vi "Manage Devices.vi"(0 "Devices queue":refnum<queue>, 1 "Table Ref In":refnum<vi>, 2 "DevNums In":i32[](array[numeric]), 3 "Col array in":refnum<class "Column.lvclass">[](array[class]), 4 "Table History ref":refnum<vi>, 5 "Layout ref":refnum<vi>) -> (7 "Devices queue out":refnum<queue>, 8 "Changes Made?":bool, 9 "DevNums Out":i32[](array[numeric]), 10 "Col array out":refnum<class "Column.lvclass">[](array[class]))   [LabVIEW 2013]
doc: "Add or Edit devices included in SetList table. Use this dialog to change SetList appearance (Column Name, Width, Colors) Trigger Line, Communication Port, etc...\nThis VI requires read/write access to Col array data."
uses:
  Device/Device.lvclass
  TypeDefs/AddDeviceRing.ctl
  ColumnVIs/Column/Column.lvclass
  TypeDefs/TableHistory.ctl
  TypeDefs/TableArray.ctl
  Master Device/Master Device.lvclass
panel:
  in  "Add Device":T1 items=["Select Type...", "DDS", "Novatech", "NI Card"]
  in  "Master Device Info":T2
  in  "Done":bool
  out "Device List in":refnum<class "Device.lvclass">[](array[class])
  in  "Slave Devices":T3(array[cluster])
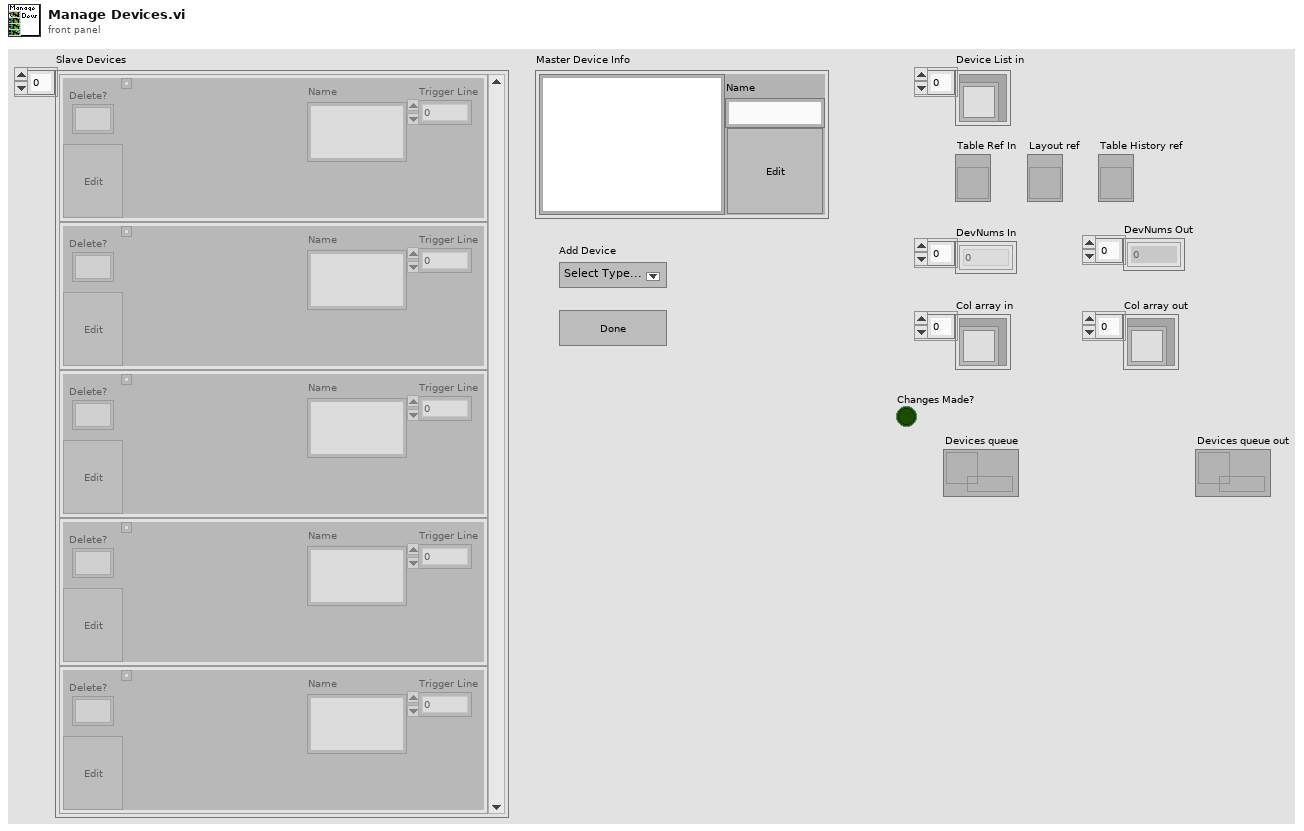
[diagram p1: front panel]
types:
  T1 = typedef "AddDeviceRing.ctl" = u16
  T2 = cluster{"2D Picture":picture, "Name":string, "Edit Device":bool}
  T3 = cluster{"Delete?":bool, "2D Picture":picture, "Name":string, "Trigger Line":i32, "Edit Device":bool}[]
  T4 = typedef "imagedata.ctl" = cluster{"image type":i32, "image depth":i32, "image":u8[], "mask":u8[], "colors":u32[], "Rectangle":cluster{"left":i16, "top":i16, "right":i16, "bottom":i16}}
  T5 = cluster{bool, "new picture":picture, "Name":string, "PB Trigger Line":u16, bool}
  T6 = cluster{"new picture":picture, "Name":string, bool}
  T7 = cluster{"Delete?":bool, "2D Picture":bool, "Name":bool, "Trigger Line":bool, "Edit Device":bool}[]
  T8 = cluster{"Delete?":bool, "2D Picture":picture, "Name":string, "Trigger Line":i32, "Edit Device":bool}
  T9 = cluster{"Delete?":bool, "new picture":picture, "Name":string, "Trigger Line":i32, "Edit Device":bool}[]
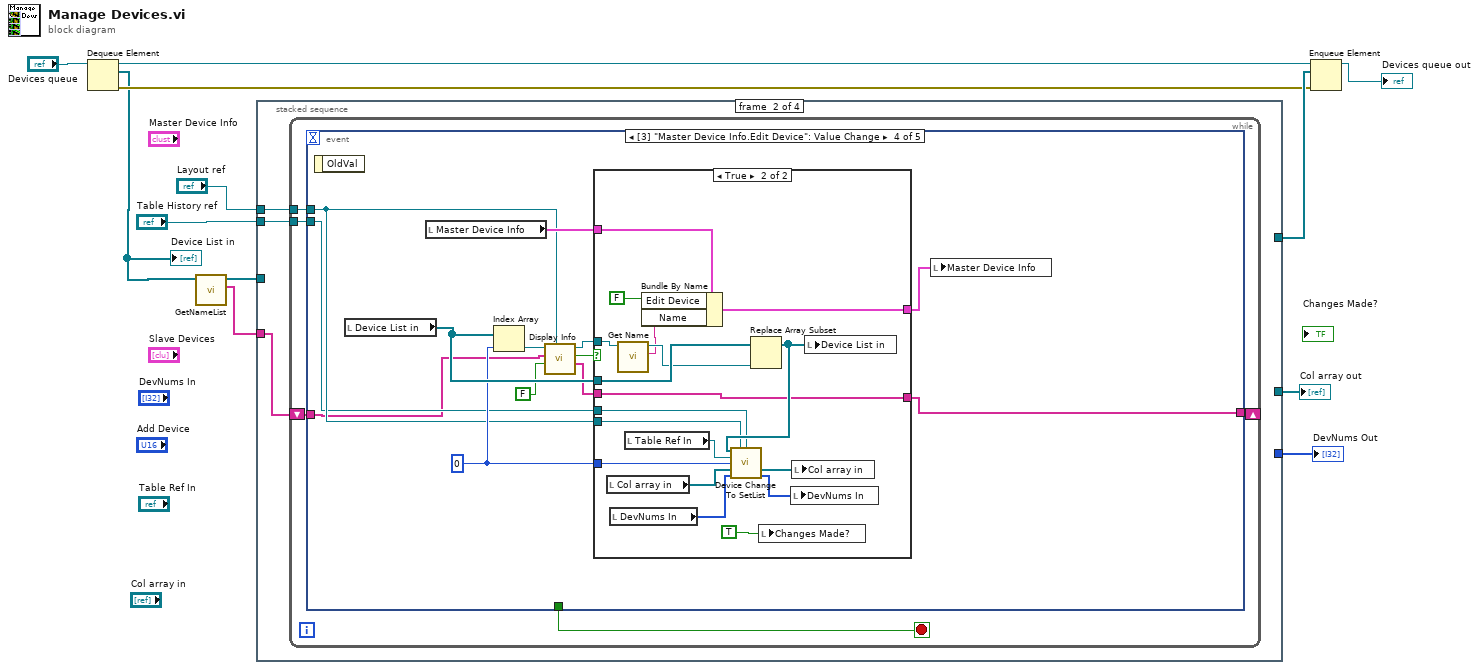
[diagram p0: block diagram]
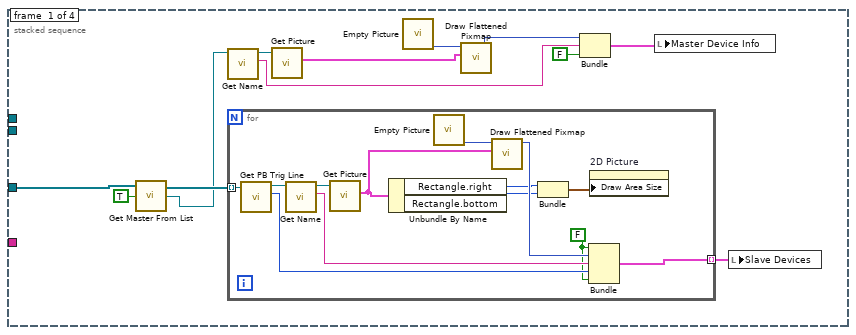
[diagram p2: hidden frame]
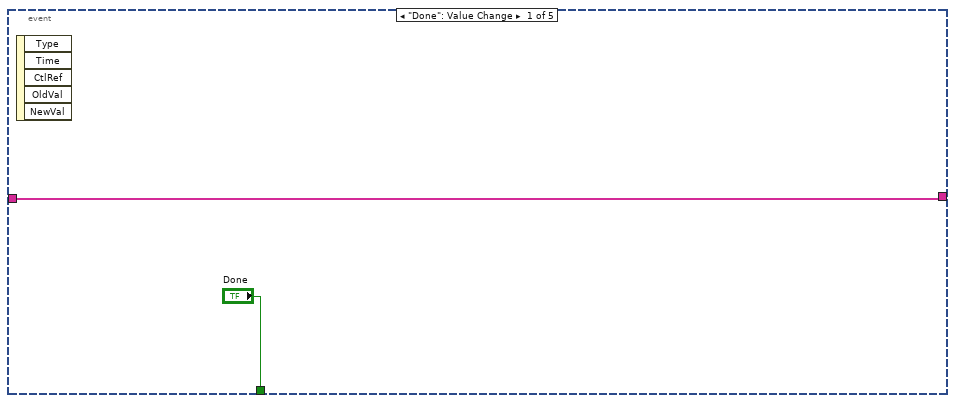
[diagram p3: hidden frame]
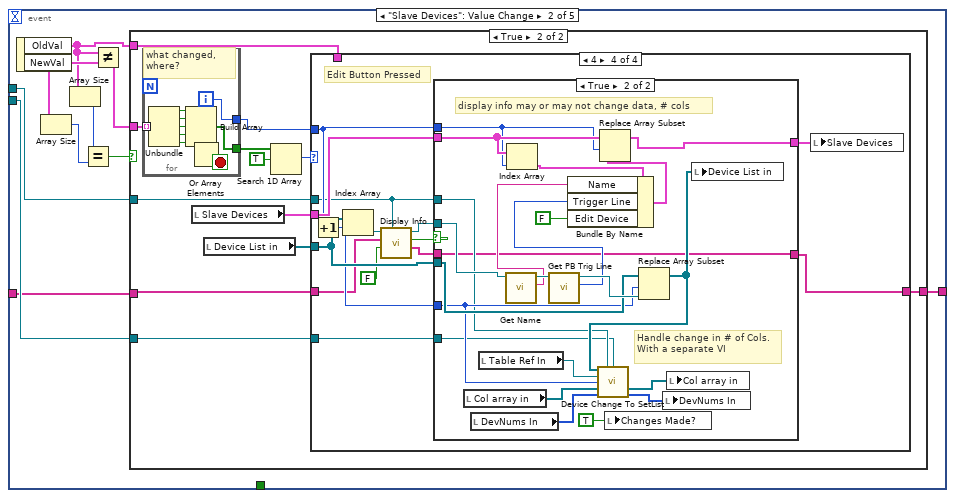
[diagram p4: hidden frame]
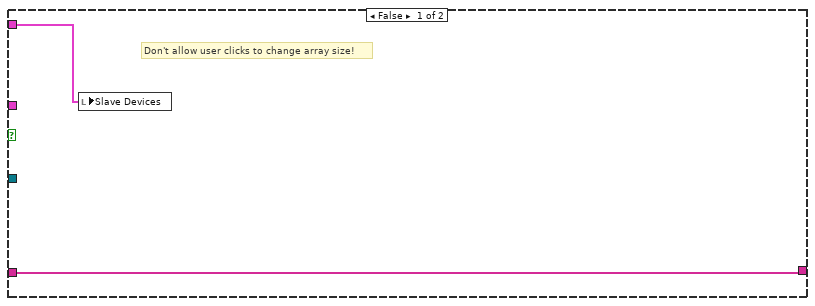
[diagram p5: hidden frame]
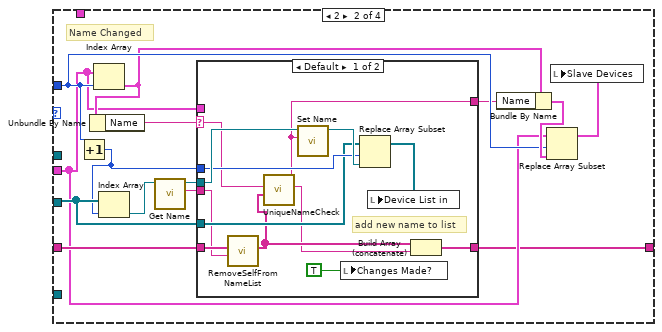
[diagram p7: hidden frame]
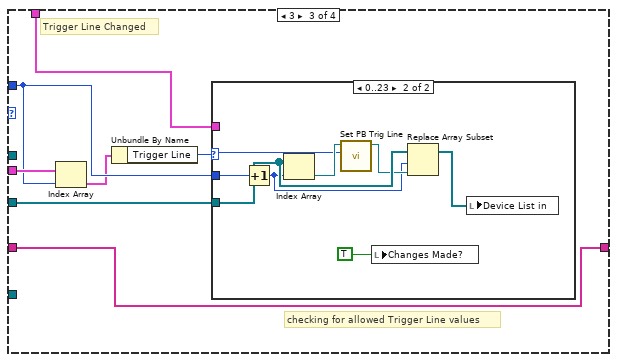
[diagram p9: hidden frame]
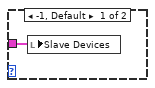
[diagram p10: hidden frame]
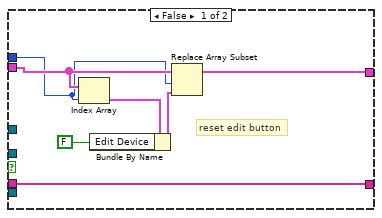
[diagram p11: hidden frame]
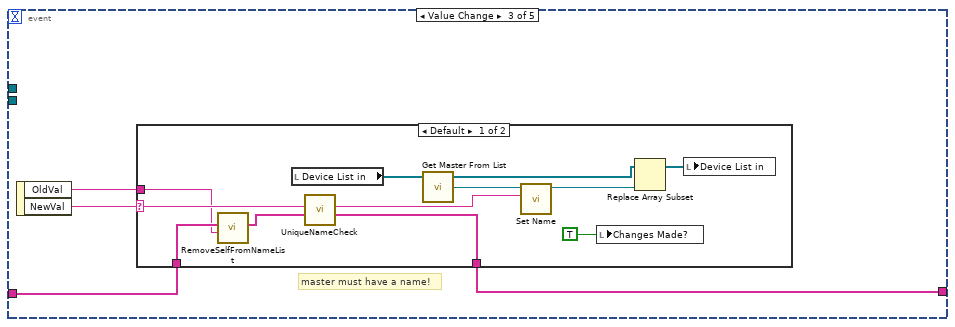
[diagram p12: hidden frame]
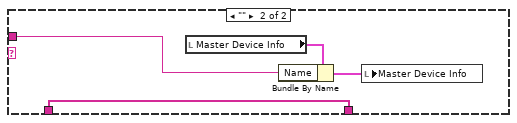
[diagram p13: hidden frame]
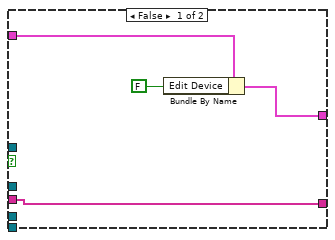
[diagram p14: hidden frame]
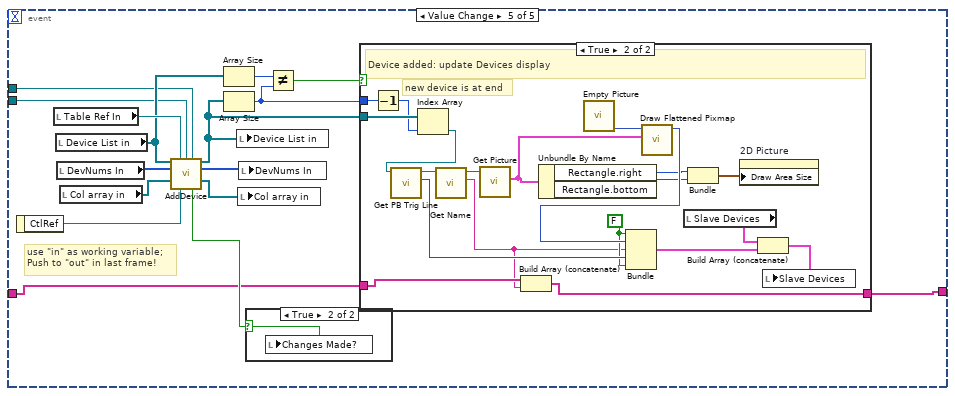
[diagram p15: hidden frame]
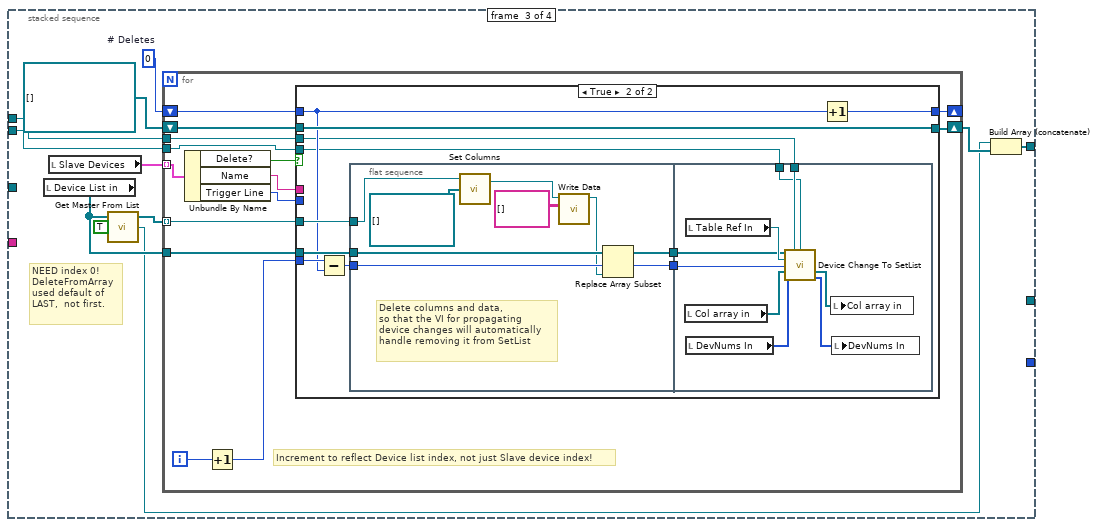
[diagram p18: hidden frame]
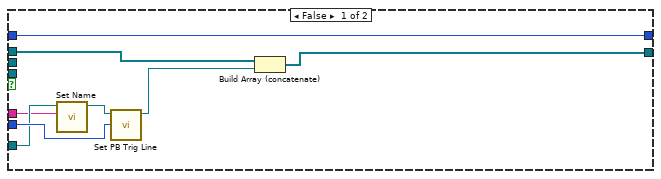
[diagram p19: hidden frame]
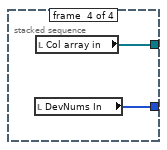
[diagram p20: hidden frame]
diagram:
  n1 = Dequeue Element(queue="Devices queue") -> (queue out=w6:refnum<queue>, element=w3:refnum<class "Device.lvclass">[], error out=w5:errorcluster)  [unwired: 2 in, 1 out]
  "Device List in" <- w3
  n2 = call "GetNameList.vi"("Devices"=w3) -> ("Names in use"=w1:string[], "Devices out"=w2:refnum<class "Device.lvclass">[])  [unwired: 8 in, 1 out]
  n3 = stacked-sequence {
    tunnel: w2 -> [w13 _ _ _]
    tunnel: [_ _ w270 _] -> w7
    tunnel: [_ _ _ w325] -> w12
    tunnel: [_ _ _ w324] -> w11
    tunnel: "Layout ref" -> [_ w40 w268 _]
    tunnel: "Table History ref" -> [_ w39 w263 _]
    tunnel: w1 -> [_ w38 _ _]
    frame #0 {
      n4 = call "Get Master From List.vi"("Del From List?"=TRUE, "Device List in"=w13) -> ("Master Device"=w14:refnum<class "Master Device.lvclass">, "Device List out"=w15:refnum<class "Device.lvclass">[])  [unwired: 1 in, 1 out]
      n5 = call-dynamic "Get Name.vi"("Device in"=w14) -> ("Name"=w18:string, "Device out"=w23:refnum<class "Master Device.lvclass">)  [unwired: 8 in, 1 out]
      n6 = for {
        tunnel: w15 -> [w37] mode=indexing
        tunnel: [w32] -> w24 mode=indexing
        w25 = FALSE
        n7 = call-dynamic "Get PB Trig Line.vi"("Device in"=w37) -> ("PB Trigger Line"=w33:u16, "Device out"=w36:refnum<class "Device.lvclass">)  [unwired: 8 in, 1 out]
        n8 = call-dynamic "Get Name.vi"("Device in"=w36) -> ("Name"=w34:string, "Device out"=w35:refnum<class "Device.lvclass">)  [unwired: 8 in, 1 out]
        n9 = call-dynamic "Get Picture.vi"("Device in"=w35) -> ("Device Pic"=w29:T4)  [unwired: 8 in, 2 out]
        n10 = Unbundle By Name(w29) -> ("Rectangle.right"=w28:i16, "Rectangle.bottom"=w27:i16)
        n11 = call "Empty Picture"() -> ("empty picture"=w31:picture)
        n12 = call <vilib>:"Draw Flattened Pixmap.vi"("image data"=w29, "picture"=w31) -> ("new picture"=w30:picture)  [unwired: 7 in]
        n13 = Bundle("right"=w28, "bottom"=w27) -> (w26:cluster{"right":i16, "bottom":i16})  [unwired: 1 in]
        n14 = Bundle(w25, "new picture"=w30, "Name"=w34, "PB Trigger Line"=w33, w25) -> (w32:T5)  [unwired: 1 in]
        n15 = property on="2D Picture" class="Pict"("Draw Area Size"=w26) -> ()  [unwired: 2 in, 2 out]
      }
      n16 = call-dynamic "Get Picture.vi"("Device in"=w23) -> ("Device Pic"=w21:T4)  [unwired: 8 in, 2 out]
      n17 = call "Empty Picture"() -> ("empty picture"=w22:picture)
      n18 = call <vilib>:"Draw Flattened Pixmap.vi"("image data"=w21, "picture"=w22) -> ("new picture"=w19:picture)  [unwired: 7 in]
      n19 = Bundle("new picture"=w19, "Name"=w18, FALSE) -> (w20:T6)  [unwired: 1 in]
      n20 = local write "Master Device Info"(w20) -> ()
      n21 = local write "Slave Devices"(w24) -> ()
    }
    frame #1 {
      n22 = while {
        tunnel: w40 -> [w44]
        tunnel: w39 -> [w43]
        shift-right: [w41] -> _
        shift-left: w38 -> [w42]
        stop <- w45 stop-if-true
        n23 = event shown="[3] \"Master Device Info.Edit Device\": Value Change" {
          selector: _ -> [_ _ _ _ _]
          dyn-events: _ -> [_ _ _ _ _]
          timeout: _ -> [_ _ _ _ _]
          tunnel: ["Done" _ _ _ _] -> w45
          tunnel: w44 -> [_ w56 _ w195 w229]
          tunnel: w43 -> [_ w55 _ w194 w227]
          tunnel: w42 -> [w46 w49 w171 w192 w226]
          tunnel: [w46 w48 w170 w191 w225] -> w41
          event "Done": Value Change {
            n24 = event-data() -> ()  [unwired: 1 in, 5 out]
          }
          event "Slave Devices": Value Change {
            n25 = event-data() -> ("OldVal"=w50:T3, "NewVal"=w54:T3)  [unwired: 1 in]
            n26 = Array Size(array=w54) -> (size(s)=w52:i32)
            n27 = Array Size(array=w50) -> (size(s)=w53:i32)
            n28 = Equal?(x=w53, y=w52) -> (x = y?=w51:bool)
            n29 = Not Equal?(x=w50, y=w54) -> (x != y?=w57:T7)
            n30 = case shown="True" w51 {
              tunnel: w57 -> [_ w71]
              tunnel: w56 -> [_ w64]
              tunnel: w55 -> [_ w63]
              tunnel: w50 -> [w59 w62]
              tunnel: w49 -> [w58 w61]
              tunnel: [w58 w60] -> w48
              frame False {
                # "Don't allow user clicks to change array size!"
                n31 = local write "Slave Devices"(w59) -> ()
              }
              frame True {
                n32 = for {
                  tunnel: w71 -> [w169] mode=indexing
                  tunnel: [w162] -> w70
                  tunnel: [w161] -> w67
                  i -> [w161]
                  stop <- w163 stop-if-true
                  # "what changed, where?"
                  n33 = Unbundle(w169) -> ("Delete?"=w168:bool, "2D Picture"=w167:bool, "Name"=w166:bool, "Trigger Line"=w165:bool, "Edit Device"=w164:bool)
                  n34 = Build Array(w168, w167, w166, w165, w164) -> (w162:bool[])
                  n35 = Or Array Elements(Boolean array=w162) -> (logical OR=w163:bool)
                }
                n36 = local read "Slave Devices"() -> (w66:T3)
                n37 = local read "Device List in"() -> (w65:refnum<class "Device.lvclass">[])
                n38 = Search 1D Array(1D array=w70, element=TRUE) -> (index of element=w68:i32)  [unwired: 1 in]
                n39 = case shown="4" w68 {
                  tunnel: w67 -> [_ w80 w105 w126]
                  tunnel: w66 -> [_ w77 w107 w127]
                  tunnel: w65 -> [_ w85 w106 w125]
                  tunnel: w64 -> [_ _ _ w122]
                  tunnel: w63 -> [_ _ _ w121]
                  tunnel: w62 -> [_ _ w102 _]
                  tunnel: w61 -> [w72 w83 w101 w119]
                  tunnel: [w72 w73 w101 w117] -> w60
                  frame 0, 1, Default {
                    # "Delete? or\nPicture Change.\n(Ignore)"
                  }
                  frame 2 {
                    # "Name Changed"
                    n40 = Increment(x=w80) -> (x+1=w84:i32)
                    n41 = Index Array(array=w77, index=w80) -> (element=w78:T8)
                    n42 = Unbundle By Name(w78) -> ("Name"=w86:string)
                    n43 = Index Array(array=w85, index=w84) -> (element=w76:refnum<class "Device.lvclass">)
                    n44 = call-dynamic "Get Name.vi"("Device in"=w76) -> ("Name"=w75:string, "Device out"=w74:refnum<class "Device.lvclass">)  [unwired: 8 in, 1 out]
                    n45 = case shown="Default" w86 {
                      selector: w86 -> [w92 _]
                      tunnel: w74 -> [w98 _]
                      tunnel: w77 -> [_ _]
                      tunnel: w84 -> [w96 _]
                      tunnel: w85 -> [w95 _]
                      tunnel: w83 -> [w91 w99]
                      tunnel: [w88 w100] -> w79
                      tunnel: w75 -> [w90 w100]
                      tunnel: [w87 w99] -> w73
                      frame Default {
                        # "add new name to list"
                        n46 = call "RemoveSelfFromNameList.vi"("self Name"=w90, "Names in use"=w91) -> ("Reserved Names"=w89:string[])  [unwired: 9 in]
                        n47 = call "UniqueNameCheck.vi"("Names in use"=w89, "Device Name"=w92) -> ("Unique name"=w88:string)  [unwired: 8 in, 1 out]
                        n48 = call-dynamic "Set Name.vi"("Name"=w88, "Device in"=w98) -> ("Device out"=w97:refnum<class "Device.lvclass">)  [unwired: 8 in, 1 out]
                        n49 = local write "Changes Made?"(TRUE ("Changes Made?")) -> ()
                        n50 = Replace Array Subset(array=w95, new element=w97, index=w96) -> (w94:refnum<class "Device.lvclass">[])
                        n51 = local write "Device List in"(w94) -> ()
                        n52 = Build Array (concatenate)(w89, w88) -> (w87:string[])
                      }
                      frame "" {
                        # "Resets the Name field if the\nuser enters an empty string"
                      }
                    }
                    n53 = Bundle By Name(cluster=w78, "Name"=w79) -> (w82:T8)
                    n54 = Replace Array Subset(array=w77, new element=w82, index=w80) -> (w81:T3)
                    n55 = local write "Slave Devices"(w81) -> ()
                  }
                  frame 3 {
                    # "checking for allowed Trigger Line values"
                    # "Trigger Line Changed"
                    n56 = Index Array(array=w107, index=w105) -> (element=w104:T8)
                    n57 = Unbundle By Name(w104) -> ("Trigger Line"=w103:i32)
                    n58 = case shown="0..23" w103 {
                      selector: w103 -> [_ w109]
                      tunnel: w106 -> [_ w116]
                      tunnel: w105 -> [_ w115]
                      tunnel: w102 -> [w108 _]
                      frame -1, Default {
                        n59 = local write "Slave Devices"(w108) -> ()
                      }
                      frame 0..23 {
                        n60 = Increment(x=w115) -> (x+1=w111:i32)
                        n61 = Index Array(array=w116, index=w111) -> (element=w114:refnum<class "Device.lvclass">)
                        n62 = call-dynamic "Set PB Trig Line.vi"("PB Trigger Line"=w109, "Device in"=w114) -> ("Device out"=w113:refnum<class "Device.lvclass">)  [unwired: 8 in, 1 out]
                        n63 = local write "Changes Made?"(TRUE ("Changes Made?")) -> ()
                        n64 = Replace Array Subset(array=w116, new element=w113, index=w111) -> (w112:refnum<class "Device.lvclass">[])
                        n65 = local write "Device List in"(w112) -> ()
                      }
                    }
                  }
                  frame 4 {
                    # "Edit Button Pressed"
                    n66 = Increment(x=w126) -> (x+1=w124:i32)
                    n67 = Index Array(array=w125, index=w124) -> (element=w130:refnum<class "Device.lvclass">)
                    n68 = call-dynamic "Display Info.vi"("Layout ref"=w122, "Modify (F) /Add [T]"=FALSE, "Names in use"=w119, "Device in"=w130) -> ("Names in use out"=w118:string[], "Changes Made?"=w129:bool, "Device out"=w128:refnum<class "Device.lvclass">)  [unwired: 4 in, 1 out]
                    n69 = case shown="True" w129 {
                      tunnel: w128 -> [_ w153]
                      tunnel: w127 -> [w137 w160]
                      tunnel: w126 -> [w135 w156]
                      tunnel: w125 -> [_ w149]
                      tunnel: w124 -> [_ w148]
                      tunnel: [w136 w154] -> w123
                      tunnel: w122 -> [_ w142]
                      tunnel: w121 -> [_ w140]
                      tunnel: [w131 w138] -> w117
                      tunnel: w118 -> [w131 w138]
                      frame False {
                        # "reset edit button"
                        n70 = Index Array(array=w137, index=w135) -> (element=w134:T8)
                        n71 = Bundle By Name(cluster=w134, "Edit Device"=FALSE) -> (w133:T8)
                        n72 = Replace Array Subset(array=w137, new element=w133, index=w135) -> (w136:T3)
                      }
                      frame True {
                        # "display info may or may not change data, # cols"
                        # "Handle change in # of Cols. With a separate VI"
                        n73 = local read "Col array in"() -> (w147:refnum<class "Column.lvclass">[])
                        n74 = local read "DevNums In"() -> (w145:i32[])
                        n75 = local read "Table Ref In"() -> (w150:refnum<vi>)
                        n76 = call-dynamic "Get Name.vi"("Device in"=w153) -> ("Name"=w139:string, "Device out"=w157:refnum<class "Device.lvclass">)  [unwired: 8 in, 1 out]
                        n77 = Index Array(array=w160, index=w156) -> (element=w159:T8)
                        n78 = call-dynamic "Get PB Trig Line.vi"("Device in"=w157) -> ("PB Trigger Line"=w152:u16, "Device out"=w155:refnum<class "Device.lvclass">)  [unwired: 8 in, 1 out]
                        n79 = Bundle By Name(cluster=w159, "Name"=w139, "Trigger Line"=w152, "Edit Device"=FALSE) -> (w158:T8)
                        n80 = Replace Array Subset(array=w160, new element=w158, index=w156) -> (w154:T3)
                        n81 = local write "Changes Made?"(TRUE ("Changes Made?")) -> ()
                        n82 = Replace Array Subset(array=w149, new element=w155, index=w148) -> (w143:refnum<class "Device.lvclass">[])
                        n83 = call "Device Change To SetList.vi"("Device List in"=w143, "Layout ref"=w142, "Table History ref"=w140, "Table Ref In"=w150, "Dev Index"=w148, "Col array in"=w147, "DevNums In"=w145) -> ("Col array out"=w146:refnum<class "Column.lvclass">[], "DevNums Out"=w144:i32[])  [unwired: 5 in, 2 out]
                        n84 = local write "DevNums In"(w144) -> ()
                        n85 = local write "Col array in"(w146) -> ()
                        n86 = local write "Device List in"(w143) -> ()
                      }
                    }
                    n87 = local write "Slave Devices"(w123) -> ()
                  }
                }
              }
            }
          }
          event "Master Device Info.Name": Value Change {
            # "master must have a name!"
            n88 = event-data() -> ("OldVal"=w172:string, "NewVal"=w173:string)  [unwired: 1 in]
            n89 = case shown="Default" w173 {
              selector: w173 -> [w179 _]
              tunnel: w172 -> [w174 w187]
              tunnel: w171 -> [w176 w186]
              tunnel: [w177 w186] -> w170
              frame Default {
                n90 = call "RemoveSelfFromNameList.vi"("self Name"=w174, "Names in use"=w176) -> ("Reserved Names"=w175:string[])  [unwired: 9 in]
                n91 = local read "Device List in"() -> (w183:refnum<class "Device.lvclass">[])
                n92 = call "UniqueNameCheck.vi"("Names in use"=w175, "Device Name"=w179) -> ("Names in use out"=w177:string[], "Unique name"=w178:string)  [unwired: 8 in]
                n93 = call "Get Master From List.vi"("Device List in"=w183) -> ("Master Device"=w182:refnum<class "Master Device.lvclass">, "Device List out"=w181:refnum<class "Device.lvclass">[])  [unwired: 2 in, 1 out]
                n94 = call-dynamic "Set Name.vi"("Name"=w178, "Device in"=w182) -> ("Device out"=w184:refnum<class "Master Device.lvclass">)  [unwired: 8 in, 1 out]
                n95 = local write "Changes Made?"(TRUE ("Changes Made?")) -> ()
                n96 = Replace Array Subset(array=w181, new element=w184) -> (w185:refnum<class "Device.lvclass">[])  [unwired: 1 in]
                n97 = local write "Device List in"(w185) -> ()
              }
              frame "" {
                n98 = local read "Master Device Info"() -> (w188:T2)
                n99 = Bundle By Name(cluster=w188, "Name"=w187) -> (w189:T2)
                n100 = local write "Master Device Info"(w189) -> ()
              }
            }
          }
          event "Master Device Info.Edit Device": Value Change {
            w197 = 0 ("Dev Index")
            n101 = event-data() -> ()  [unwired: 1 in, 1 out]
            n102 = local read "Device List in"() -> (w200:refnum<class "Device.lvclass">[])
            n103 = local read "Master Device Info"() -> (w198:T2)
            n104 = Index Array(array=w200, index=w197) -> (element=w202:refnum<class "Device.lvclass">)
            n105 = call-dynamic "Display Info.vi"("Layout ref"=w195, "Modify (F) /Add [T]"=FALSE, "Names in use"=w192, "Device in"=w202) -> ("Names in use out"=w190:string[], "Changes Made?"=w201:bool, "Device out"=w196:refnum<class "Device.lvclass">)  [unwired: 4 in, 1 out]
            n106 = case shown="True" w201 {
              tunnel: w196 -> [_ w224]
              tunnel: w200 -> [_ w223]
              tunnel: [w205 w221] -> w199
              tunnel: w198 -> [w206 w220]
              tunnel: w197 -> [_ w214]
              tunnel: w195 -> [_ w211]
              tunnel: w194 -> [_ w209]
              tunnel: w190 -> [w203 w207]
              tunnel: [w203 w207] -> w191
              frame False {
                n107 = Bundle By Name(cluster=w206, "Edit Device"=FALSE) -> (w205:T2)
              }
              frame True {
                n108 = local read "Col array in"() -> (w215:refnum<class "Column.lvclass">[])
                n109 = local read "DevNums In"() -> (w212:i32[])
                n110 = call-dynamic "Get Name.vi"("Device in"=w224) -> ("Name"=w208:string, "Device out"=w222:refnum<class "Device.lvclass">)  [unwired: 8 in, 1 out]
                n111 = local read "Table Ref In"() -> (w218:refnum<vi>)
                n112 = Bundle By Name(cluster=w220, "Edit Device"=FALSE, "Name"=w208) -> (w221:T2)
                n113 = Replace Array Subset(array=w223, new element=w222) -> (w217:refnum<class "Device.lvclass">[])  [unwired: 1 in]
                n114 = call "Device Change To SetList.vi"("Device List in"=w217, "Layout ref"=w211, "Table History ref"=w209, "Table Ref In"=w218, "Dev Index"=w214, "Col array in"=w215, "DevNums In"=w212) -> ("Col array out"=w216:refnum<class "Column.lvclass">[], "DevNums Out"=w213:i32[])  [unwired: 5 in, 2 out]
                n115 = local write "Changes Made?"(TRUE ("Changes Made?")) -> ()
                n116 = local write "DevNums In"(w213) -> ()
                n117 = local write "Col array in"(w216) -> ()
                n118 = local write "Device List in"(w217) -> ()
              }
            }
            n119 = local write "Master Device Info"(w199) -> ()
          }
          event Value Change {
            # "use \"in\" as working variable;\nPush to \"out\" in last frame!"
            n120 = event-data() -> ("CtlRef"=w240:refnum<vi>)  [unwired: 1 in]
            n121 = local read "Table Ref In"() -> (w235:refnum<vi>)
            n122 = local read "Device List in"() -> (w234:refnum<class "Device.lvclass">[])
            n123 = local read "DevNums In"() -> (w239:i32[])
            n124 = local read "Col array in"() -> (w237:refnum<class "Column.lvclass">[])
            n125 = call "AddDevice.vi"("Device List in"=w234, "Table Ref In"=w235, "Table History ref"=w227, "Layout Ref"=w229, "DevNums In"=w239, "Col array in"=w237, "Add Device"=w240) -> ("Device List out"=w231:refnum<class "Device.lvclass">[], "DevNums Out"=w238:i32[], "Col array out"=w236:refnum<class "Column.lvclass">[], "Changes Made?"=w228:bool)  [unwired: 4 in, 1 out]
            n126 = Array Size(array=w234) -> (size(s)=w233:i32)
            n127 = Array Size(array=w231) -> (size(s)=w230:i32)
            n128 = local write "Device List in"(w231) -> ()
            n129 = local write "Col array in"(w236) -> ()
            n130 = local write "DevNums In"(w238) -> ()
            n131 = case shown="True" w228 {
              selector: w228 -> [_ w241]
              frame False {
              }
              frame True {
                n132 = local write "Changes Made?"(w241) -> ()
              }
            }
            n133 = Not Equal?(x=w233, y=w230) -> (x != y?=w232:bool)
            n134 = case shown="True" w232 {
              tunnel: w231 -> [_ w252]
              tunnel: w230 -> [_ w250]
              tunnel: w226 -> [w242 w245]
              tunnel: [w242 w243] -> w225
              frame False {
              }
              frame True {
                w253 = FALSE
                # "new device is at end"
                # "Device added: update Devices display"
                n135 = Decrement(x=w250) -> (x-1=w249:i32)
                n136 = Index Array(array=w252, index=w249) -> (element=w251:refnum<class "Device.lvclass">)
                n137 = call-dynamic "Get PB Trig Line.vi"("Device in"=w251) -> ("PB Trigger Line"=w260:u16, "Device out"=w262:refnum<class "Device.lvclass">)  [unwired: 8 in, 1 out]
                n138 = call-dynamic "Get Name.vi"("Device in"=w262) -> ("Name"=w244:string, "Device out"=w261:refnum<class "Device.lvclass">)  [unwired: 8 in, 1 out]
                n139 = call-dynamic "Get Picture.vi"("Device in"=w261) -> ("Device Pic"=w257:T4)  [unwired: 8 in, 2 out]
                n140 = Build Array (concatenate)(w245, w244) -> (w243:string[])
                n141 = Unbundle By Name(w257) -> ("Rectangle.right"=w256:i16, "Rectangle.bottom"=w255:i16)
                n142 = call "Empty Picture"() -> ("empty picture"=w259:picture)
                n143 = call <vilib>:"Draw Flattened Pixmap.vi"("image data"=w257, "picture"=w259) -> ("new picture"=w258:picture)  [unwired: 7 in]
                n144 = Bundle(w253, "new picture"=w258, "Name"=w244, "PB Trigger Line"=w260, w253) -> (w247:T5)  [unwired: 1 in]
                n145 = local read "Slave Devices"() -> (w248:T3)
                n146 = Bundle("right"=w256, "bottom"=w255) -> (w254:cluster{"right":i16, "bottom":i16})  [unwired: 1 in]
                n147 = property on="2D Picture" class="Pict"("Draw Area Size"=w254) -> ()  [unwired: 2 in, 2 out]
                n148 = Build Array (concatenate)(w248, w247) -> (w246:T9)
                n149 = local write "Slave Devices"(w246) -> ()
              }
            }
          }
        }
      }
    }
    frame #2 {
      w269 = 0  # # Deletes
      # "NEED index 0!\nDeleteFromArray\nused default of\nLAST,  not first."
      n150 = local read "Device List in"() -> (w266:refnum<class "Device.lvclass">[])
      n151 = local read "Slave Devices"() -> (w273:T3)
      n152 = call "Get Master From List.vi"("Del From List?"=TRUE, "Device List in"=w266) -> ("Master Device"=w265:refnum<class "Master Device.lvclass">, "Device List out"=w267:refnum<class "Device.lvclass">[])  [unwired: 1 in, 1 out]
      n153 = for {
        tunnel: w273 -> [w287] mode=indexing
        shift-right: [w284] -> w271
        shift-left: refnum<class "Device.lvclass">[] [] ("Device List in") -> [w285]
        tunnel: w267 -> [w283] mode=indexing
        tunnel: w266 -> [w280]
        shift-right: [w276] -> _
        shift-left: w269 -> [w277]
        tunnel: w268 -> [w275]
        tunnel: w263 -> [w274]
        i -> [w279]
        # "Increment to reflect Device list index, not just Slave device index!"
        n154 = Unbundle By Name(w287) -> ("Delete?"=w286:bool, "Name"=w281:string, "Trigger Line"=w282:i32)
        n155 = Increment(x=w279) -> (x+1=w278:i32)
        n156 = case shown="True" w286 {
          tunnel: [w294 w306] -> w284
          tunnel: w285 -> [w295 w306]
          tunnel: w283 -> [w291 w305]
          tunnel: w282 -> [w293 _]
          tunnel: w281 -> [w290 _]
          tunnel: w280 -> [_ w304]
          tunnel: w278 -> [_ w300]
          tunnel: w277 -> [w288 w299]
          tunnel: [w288 w301] -> w276
          tunnel: w275 -> [_ w297]
          tunnel: w274 -> [_ w296]
          frame False {
            n157 = call-dynamic "Set Name.vi"("Name"=w290, "Device in"=w291) -> ("Device out"=w292:refnum<class "Device.lvclass">)  [unwired: 8 in, 1 out]
            n158 = call-dynamic "Set PB Trig Line.vi"("PB Trigger Line"=w293, "Device in"=w292) -> ("Device out"=w289:refnum<class "Device.lvclass">)  [unwired: 8 in, 1 out]
            n159 = Build Array (concatenate)(w295, w289) -> (w294:refnum<class "Device.lvclass">[])
          }
          frame True {
            n160 = Subtract(x=w300, y=w299) -> (x-y=w298:i32)
            n161 = flat-sequence {
              tunnel: w305 -> [w312]
              tunnel: w304 -> [w310]
              tunnel: w298 -> [w309]
              tunnel: [w309] -> w303
              tunnel: [w307] -> w302
              tunnel: w303 -> [w317]
              tunnel: w302 -> [w318]
              tunnel: w297 -> [w316]
              tunnel: w296 -> [w315]
              frame #0 {
                # "Delete columns and data,\nso that the VI for propagating\ndevice changes will automatically\nhandle removing it from SetList"
                n162 = call-dynamic "Set Columns.vi"("Columns"=refnum<class "Column.lvclass">[] [], "Device in"=w312) -> ("Device out"=w313:refnum<class "Device.lvclass">)  [unwired: 2 in, 1 out]
                n163 = call-dynamic "Write Data.vi"("Data"=string[][] [], "Device in"=w313) -> ("Device Out"=w308:refnum<class "Device.lvclass">)  [unwired: 8 in, 1 out]
                n164 = Replace Array Subset "Replace Array Subset"(array=w310, new element=w308, index=w309) -> (w307:refnum<class "Device.lvclass">[])
              }
              frame #1 {
                n165 = local read "Col array in"() -> (w322:refnum<class "Column.lvclass">[])
                n166 = local read "Table Ref In"() -> (w323:refnum<vi>)
                n167 = local read "DevNums In"() -> (w319:i32[])
                n168 = call "Device Change To SetList.vi"("Device List in"=w318, "Layout ref"=w316, "Table History ref"=w315, "Table Ref In"=w323, "Dev Index"=w317, "Col array in"=w322, "DevNums In"=w319) -> ("Col array out"=w321:refnum<class "Column.lvclass">[], "DevNums Out"=w320:i32[])  [unwired: 5 in, 2 out]
                n169 = local write "Col array in"(w321) -> ()
                n170 = local write "DevNums In"(w320) -> ()
              }
            }
            n171 = Increment(x=w299) -> (x+1=w301:i32)
          }
        }
      }
      n172 = Build Array (concatenate)(w265, w271) -> (w270:refnum<class "Device.lvclass">[])
    }
    frame #3 {
      n173 = local read "DevNums In"() -> (w324:i32[])
      n174 = local read "Col array in"() -> (w325:refnum<class "Column.lvclass">[])
    }
  }
  "DevNums Out" <- w11
  "Col array out" <- w12
  n175 = Enqueue Element(queue=w6, element=w7, error in (no error)=w5) -> (queue out=→"Devices queue out":refnum<queue>)  [unwired: 1 in, 2 out]
